vi "connect.vi"(6 "timeout":i32=30, 8 "error in":errorcluster, 9 "password":string, 10 "username":string="notuniqueuser", 11 "MQTT client in":refnum<class "MQTT client.lvclass">) -> (0 "error out":errorcluster, 3 "MQTT client out":refnum<class "MQTT client.lvclass">)   [LabVIEW 2014, in "MQTT client.lvclass"]
uses:
  MQTT client.lvclass
  MQTT client.lvclass/MQTT client.ctl
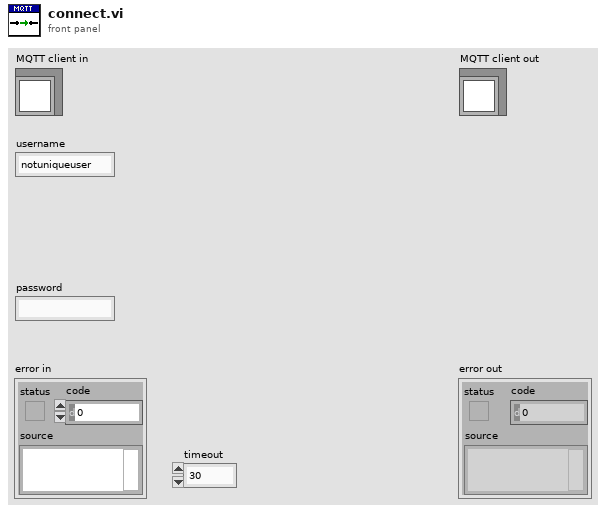
[diagram p1: front panel]
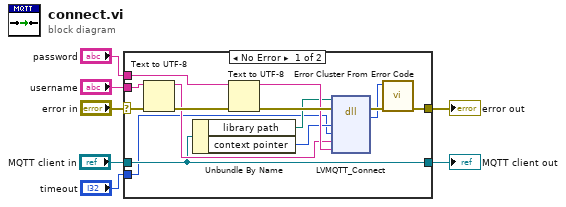
[diagram p0: block diagram]
diagram:
  n1 = case shown="No Error" "error in" {
    selector: "error in" -> [w15 w23]
    tunnel: [w14 w23] -> w6
    tunnel: [w13 w22] -> w4
    tunnel: "MQTT client in" -> [w13 w22]
    tunnel: "timeout" -> [w10 _]
    tunnel: "username" -> [w9 _]
    tunnel: "password" -> [w8 _]
    frame No Error {
      n2 = Text to UTF-8(8:w15, 11:w9) -> (0:w19:errorcluster, 3:w16:string)  [unwired: 1 in]
      n3 = Unbundle By Name(w13) -> ("library path"=w11:path, "context pointer"=w12:u64)
      n4 = Text to UTF-8(8:w19, 11:w8) -> (0:w18:errorcluster, 3:w17:string)  [unwired: 1 in]
      n5 = dll-call lib="paho-mqtt3a.*" fn="LVMQTT_Connect"(path in=w11, error in=w18, "lvctx"=w12, "timeout"=w10, "uname"=w16, "pass"=w17) -> (error out=w21:errorcluster, "return type"=w20:i32)  [unwired: 5 in, 1 out]
      n6 = call <vilib>:"Error Cluster From Error Code.vi"("error in (no error)"=w21, "error code (0)"=w20) -> ("error out"=w14:errorcluster)  [unwired: 7 in]
    }
    frame Error {
    }
  }
  "error out" <- w6
  "MQTT client out" <- w4
